vi "Load Aborts from XML.vi"(8 "error in (no error)":errorcluster, 11 "Abort Parameters In":T1 {"Abort Criteria"."Comparison" items=["<", ">"]}) -> (0 "error out":errorcluster, 3 "Abort Parameters Out":T1 {"Abort Criteria"."Comparison" items=["<", ">"]})   [LabVIEW 2024]
doc: "Attempts to load previous user specified settings from an XML file.\n\nThis VI will not generate an error. If a suitable XML file can't be loaded and parsed then it will simply return the default settings."
uses:
  Abort Parameters.ctl
  <vilib>/Utility/xml.llb/Read From XML File(string).vi
  <vilib>/Utility/xml.llb/Write to XML File(string).vi
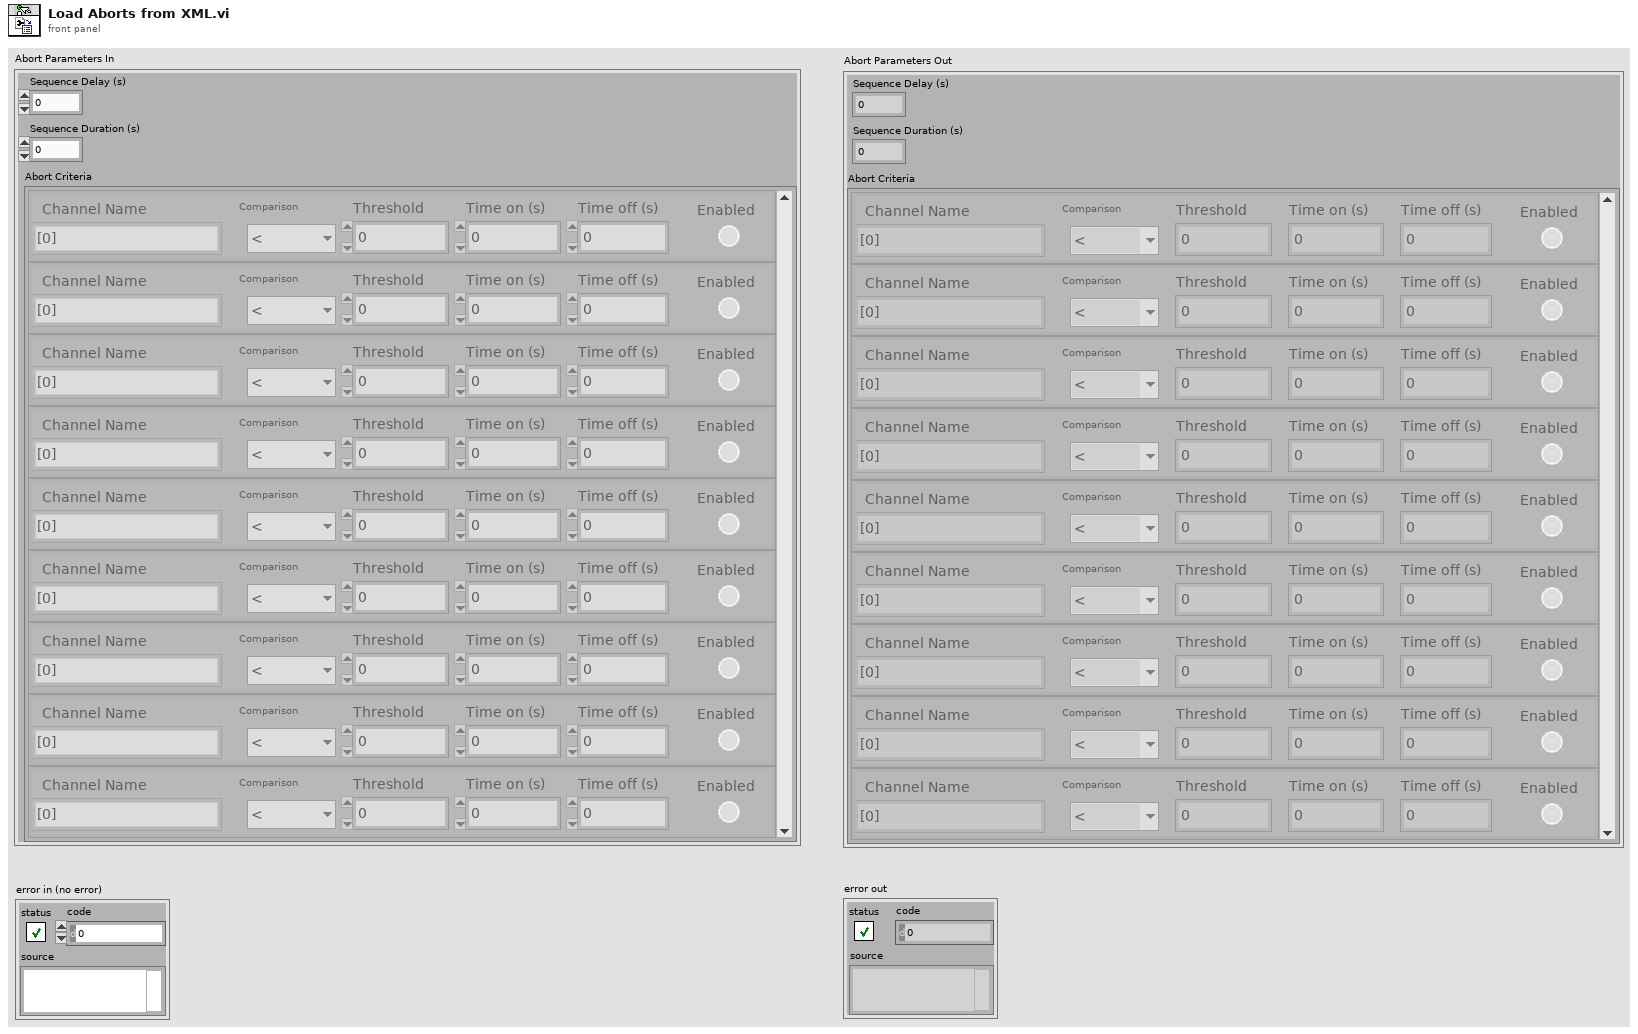
[diagram p1: front panel]
types:
  T1 = typedef "Abort Parameters.ctl" = cluster{"Sequence Delay (s)":dbl, "Sequence Duration (s)":dbl, "Abort Criteria":cluster{"Channel Name\n":enum16{"[0]", "[1]", "[2]", "[3]", "[4]", "[5]", "[6]", "[7]", "[8]", "[9]", "[10]", "[11]", "[12]", "[13]", "[14]", "[15]", "[16]", "[17]", "[18]", "[19]", "[20]", "[21]", "[22]", "[23]", "[24]", "[25]", "[26]", "[27]", "[28]", "[29]", "[30]", "[31]", "[32]", "[33]", "[34]", "[35]", "[36]", "[37]", "[38]", "[39]", "[40]", "[41]", "[42]", "[43]", "[44]", "[45]", "[46]", "[47]", "[48]", "[49]"}, "Comparison\n":u16, "Threshold":dbl, "Time on (s)":dbl, "Time off (s)":dbl, "Enabled":bool}[]}
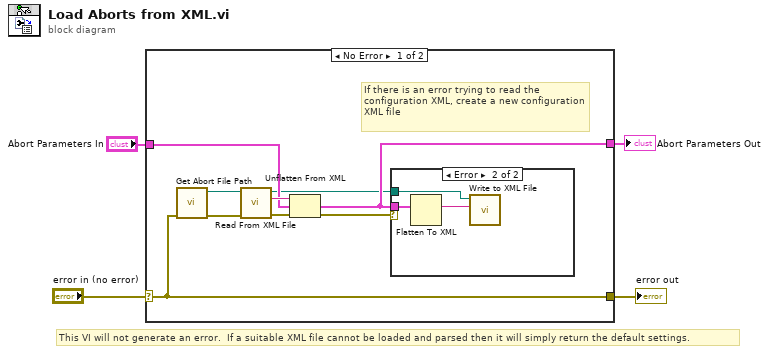
[diagram p0: block diagram]
diagram:
  # "This VI will not generate an error.  If a suitable XML file cannot be loaded and parsed then it will simply return the default settings."
  n1 = case shown="No Error" "error in (no error)" {
    selector: "error in (no error)" -> [w7 w17]
    tunnel: [w7 w17] -> w3
    tunnel: "Abort Parameters In" -> [w9 w16]
    tunnel: [w8 w16] -> w1
    frame No Error {
      # "If there is an error trying to read the configuration XML, create a new configuration XML file"
      n2 = call "Get Abort File Path.vi"("error in (no error)"=w7) -> ("error out"=w5:errorcluster, "XML File Path"=w6:path)  [unwired: 9 in]
      n3 = call-poly <vilib>:"Read From XML File.vi"("error in (no error)"=w5, "XML File Path"=w6) -> ("error out"=w11:errorcluster, "XML Elements"=w12:string)  [unwired: 7 in, 1 out]
      n4 = Unflatten From XML(xml string=w12, type=w9, error in (no error)=w11) -> (value=w8:T1, error out=w10:errorcluster)
      n5 = case shown="Error" w10 {
        tunnel: w8 -> [_ w15]
        tunnel: w6 -> [_ w13]
        frame No Error {
        }
        frame Error {
          n6 = Flatten To XML(6:w15) -> (2:w14:string)
          n7 = call-poly <vilib>:"Write to XML File.vi"("XML Input"=w14, "XML File Path"=w13) -> ()  [unwired: 7 in, 3 out]
        }
      }
    }
    frame Error {
    }
  }
  "error out" <- w3
  "Abort Parameters Out" <- w1
